vi "sv_Maximum Harmonic to Samples per Rev.vi"(10 "maximum harmonic":i32) -> (2 "samples/rev":i32)   [LabVIEW 2017, in "SoundVib_ContSweptSine.lvlib"]
uses:
  <vilib>/addons/Sound and Vibration/svt_Continuous Swept Sine/SoundVib_ContSweptSine.lvlib
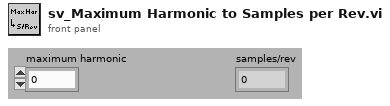
[diagram p1: front panel]
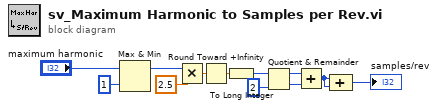
[diagram p0: block diagram]
diagram:
  n1 = Max & Min(x="maximum harmonic", y=1) -> (max(x,y)=w3:i32)  [unwired: 1 out]
  n2 = Multiply(x=w3, y=2.5) -> (x*y=w11:dbl)
  n3 = Round Toward +Infinity(x=w11) -> (ceil(x): smallest int >= x=w10:dbl)
  n4 = To Long Integer(number=w10) -> (32bit integer=w5:i32)
  n5 = Quotient & Remainder(x=w5, y=2) -> (x-y*floor(x/y)=w8:i32, floor(x/y)=w7:i32)
  n6 = Add(x=w8, y=w7) -> (x+y=w6:i32)
  n7 = Compound Arithmetic op=ADD(w6, w6) -> (→"samples/rev":i32)
